vi "initialise.vi"(8 "error in (no error)":errorcluster, 11 "GenericPlugin in":refnum<class "StageFH090410SharedVariable.lvclass">) -> (0 "error out":errorcluster, 3 "GenericPlugin out":refnum<class "StageFH090410SharedVariable.lvclass">)   [LabVIEW 2010, in "StageFH090410SharedVariable.lvclass"]
doc: "The dynamic dispatch-version of this VI initalises the plug-in object by allocating and initalising any dynamic resources need."
uses:
  StageFH090410SharedVariable.lvclass
  StageDL090409Scaffold/StageDL090409Scaffold/StageDL090409Scaffold.lvclass
  ControllerSimulator/space_vector_cluster.ctl
  StageFH090410SharedVariable.lvclass/StageFH090410SharedVariable.ctl
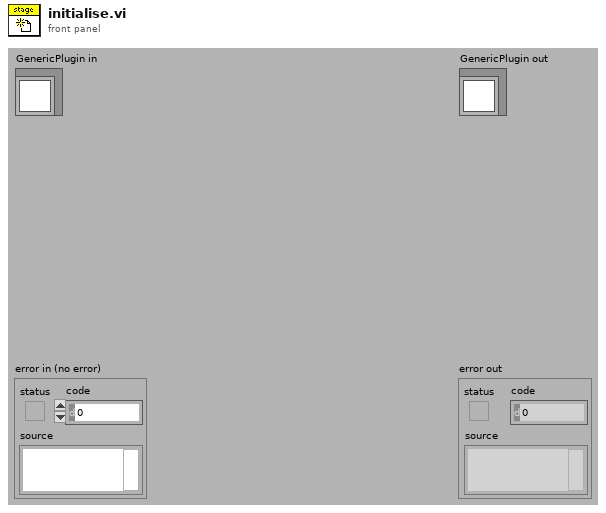
[diagram p1: front panel]
types:
  T1 = typedef "space_vector_cluster.ctl" = cluster{"x":dbl[unit], "y":dbl[unit], "z":dbl[unit]}
  T2 = typedef "StageFH090410SharedVariable.lvclass/command_mode_enum.ctl" = enum16{"step", "absolute"}
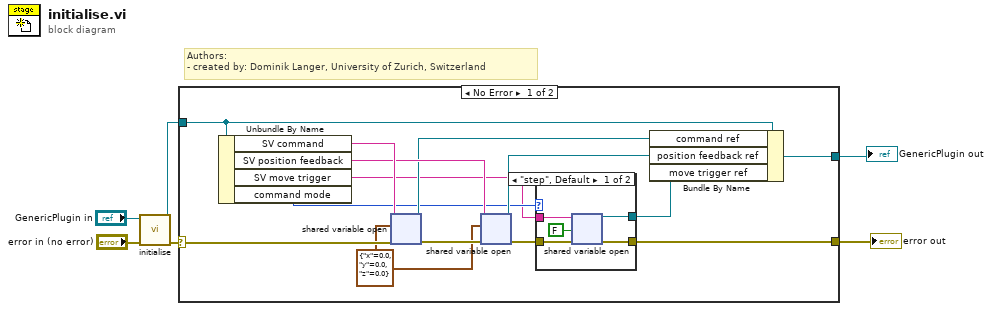
[diagram p0: block diagram]
diagram:
  # "Authors: \n- created by: Dominik Langer, University of Zurich, Switzerland"
  n1 = call-parent "initialise.vi"("error in (no error)"="error in (no error)", "GenericPlugin in"="GenericPlugin in") -> ("error out"=w4:errorcluster, "GenericPlugin out"=w3:refnum<class "StageFH090410SharedVariable.lvclass">)  [unwired: 8 in]
  n2 = case shown="No Error" w4 {
    selector: w4 -> [w19 w27]
    tunnel: w3 -> [w14 w26]
    tunnel: [w15 w27] -> w2
    tunnel: [w7 w26] -> w1
    frame No Error {
      w12 = T1 {"x"=0.0, "y"=0.0, "z"=0.0} ("space vector")
      n3 = Unbundle By Name(w14) -> ("SV command"=w18:string, "SV position feedback"=w17:string, "SV move trigger"=w8:string, "command mode"=w9:T2)
      n4 = shared-variable-open(w18, w19, w12) -> (w11:refnum<k21>, w16:errorcluster)  [unwired: 1 in]
      n5 = shared-variable-open(w17, w16, w12) -> (w13:refnum<k21>)  [unwired: 1 in, 1 out]
      n6 = case shown="\"step\", Default" w9 {
        tunnel: w8 -> [w24 _]
        tunnel: w16 -> [w23 w25]
        tunnel: [w22 w25] -> w15
        tunnel: [w20 _] -> w10
        frame "step", Default {
          n7 = shared-variable-open(w24, w23, FALSE) -> (w20:refnum<k21>, w22:errorcluster)  [unwired: 1 in]
        }
        frame "absolute" {
        }
      }
      n8 = Bundle By Name(cluster=w14, "command ref"=w11, "position feedback ref"=w13, "move trigger ref"=w10) -> (w7:refnum<class "StageFH090410SharedVariable.lvclass">)
    }
    frame Error {
    }
  }
  "error out" <- w2
  "GenericPlugin out" <- w1
